vi "Main.vi"() -> ()   [LabVIEW 2018] (continued)
                n2991 = call "S7_Read.vi"("TCP"=w2079, "DB #"=u16 20, "读取长度"=u16 13, "寄存器类型"=w2083, "起始地址"=u32 82, "数据类型"=w2081, "error in"=w2078) -> ("TCP"=w2077:refnum<k5>, "数据"=w2086:u32[], "error out"=w2088:errorcluster)  [unwired: 5 in, 1 out]
                n2992 = To Unsigned Word Integer(number=w2086) -> (unsigned 16bit integer=w2087:u16[])
                n2993 = call "还原为字符串.vi"("error in (no error)"=w2088, "输入数组"=w2087) -> ("error out"=w2076:errorcluster, "字符串"=w2080:string)  [unwired: 8 in]
                n2994 = call "S7_Read.vi"("TCP"=w2077, "DB #"=u16 20, "读取长度"=u16 2, "寄存器类型"=w2105, "起始地址"=u32 212, "数据类型"=w2107, "error in"=w2076) -> ("TCP"=w2101:refnum<k5>, "数据"=w2100:u32[], "error out"=w2102:errorcluster)  [unwired: 5 in, 1 out]
                n2995 = Index Array(array=w2100) -> (element #1=w2099:u32, element #2=w2095:u32)  [unwired: 2 in]
                n2996 = Equal?(x=w2095, y=u32 1) -> (x = y?=w2096:bool)
                n2997 = Equal?(x=w2099, y=u32 1) -> (x = y?=w2094:bool)
                n2998 = call "S7_Read.vi"("TCP"=w2101, "DB #"=u16 20, "读取长度"=u16 1, "寄存器类型"=w2111, "起始地址"=u32 136, "数据类型"=w2109, "error in"=w2102) -> ("TCP"=w2125:refnum<k5>, "数据"=w2127:u32[], "error out"=w2126:errorcluster)  [unwired: 5 in, 1 out]
                n2999 = case shown="真" w2096 {
                  tunnel: ["NG" "OK"] -> w2092
                  frame False {
                  }
                  frame True {
                  }
                }
                n3000 = case shown="真" w2094 {
                  tunnel: ["NG" "OK"] -> w2093
                  frame False {
                  }
                  frame True {
                  }
                }
                n3001 = local write "503二维码"(w2080) -> ()
                n3002 = call "S7_Read.vi"("TCP"=w2125, "DB #"=u16 20, "读取长度"=u16 1, "寄存器类型"=w2116, "起始地址"=u32 128, "数据类型"=w2114, "error in"=w2126) -> ("TCP"=w2108:refnum<k5>, "数据"=w2129:u32[], "error out"=w2091:errorcluster)  [unwired: 5 in, 1 out]
                n3003 = Index Array(array=w2127) -> (element=w2128:u32)  [unwired: 1 in]
                n3004 = Number To Decimal String(number=w2128) -> (decimal integer string=w2135:string)  [unwired: 1 in]
                n3005 = Index Array(array=w2129) -> (element=w2131:u32)  [unwired: 1 in]
                n3006 = Equal?(x=w2131, y=u32 1) -> (x = y?=w2130:bool)
                n3007 = case shown="真" w2130 {
                  tunnel: ["NG" "OK"] -> w2134
                  frame False {
                  }
                  frame True {
                  }
                }
                n3008 = Format Date/Time String(time format string (%c)="%Y-%m-%d" ("时间格式字符串(%c)")) -> (date/time string=w2132:string)  [unwired: 2 in]
                n3009 = Get Date/Time String(want seconds? (F)=TRUE ("需要秒？(F)")) -> (time string=w2133:string)  [unwired: 2 in, 1 out]
                n3010 = Insert Into Array(array=string[] [] ("数组"), index=0 ("索引"), new element #1="503" ("新元素/子数组"), new element #2=w2134, new element #3=w2132, new element #4=w2133, new element #5=w2134, new element #6=w2135, new element #7=w2093, new element #8=w2092) -> (w2089:string[])
                n3011 = stacked-sequence {
                  tunnel: w2091 -> [_ w2139]
                  tunnel: [_ w2138] -> w2090
                  tunnel: w2089 -> [w2136 _]
                  frame #0 {
                    "503data" <- w2136
                  }
                  frame #1 {
                    n3012 = property on="ST503数据读取（事件）" class="Bool (严格)"(error in=w2139, "Val(Sgnl)"=TRUE ("值(信号)")) -> (error out=w2138:errorcluster)  [unwired: 1 in, 1 out]
                  }
                }
              }
            }
            n3013 = call <vilib>:"Boolean Crossing PtByPt.vi"("direction"=enum16{"either", "false-true", "true-false"}."false-true", "input"=w1819) -> ("crossing"=w1830:bool)  [unwired: 1 in]
            n3014 = case shown="真" w1830 {
              tunnel: w1829 -> [w2052 w2058]
              tunnel: w1828 -> [w2051 w2057]
              tunnel: [w2051 w2054] -> w1827
              tunnel: [w2052 w2056] -> w1826
              frame False {
              }
              frame True {
                w2059 = u16 0 items=["byte", "word", "Dword"] ("数据类型")
                w2061 = u8 132 items=["I/O (P)"=128, "Input (I)"=129, "Output (Q)"=130, "Bit Memory (M)"=131, "Data (DB)"=132, "Instance Data (DI)"=133, "Local Data (L)"=134, "Predecessor Local Data (VL)"=135] ("寄存器类型")
                # "原82"
                n3015 = call "S7_Read.vi"("TCP"=w2058, "DB #"=u16 20, "读取长度"=u16 13, "寄存器类型"=w2061, "起始地址"=u32 104, "数据类型"=w2059, "error in"=w2057) -> ("TCP"=w2056:refnum<k5>, "数据"=w2064:u32[], "error out"=w2066:errorcluster)  [unwired: 5 in, 1 out]
                n3016 = To Unsigned Word Integer(number=w2064) -> (unsigned 16bit integer=w2065:u16[])
                n3017 = call "还原为字符串.vi"("error in (no error)"=w2066, "输入数组"=w2065) -> ("error out"=w2055:errorcluster, "字符串"=w2053:string)  [unwired: 8 in]
                n3018 = stacked-sequence {
                  tunnel: w2055 -> [_ w2070]
                  tunnel: [_ w2069] -> w2054
                  tunnel: w2053 -> [w2067 _]
                  frame #0 {
                    "504二维码" <- w2067
                  }
                  frame #1 {
                    n3019 = property on="ST504扫码请求（事件）" class="Bool (严格)"(error in=w2070, "Val(Sgnl)"=TRUE ("值(信号)")) -> (error out=w2069:errorcluster)  [unwired: 1 in, 1 out]
                  }
                }
              }
            }
            n3020 = call <vilib>:"Boolean Crossing PtByPt.vi"("direction"=enum16{"either", "false-true", "true-false"}."false-true", "input"=w1818) -> ("crossing"=w1824:bool)  [unwired: 1 in]
            n3021 = case shown="真" w1824 {
              tunnel: w1826 -> [w1919 w1923]
              tunnel: w1827 -> [w1918 w1922]
              tunnel: [w1919 w2009] -> w1823
              tunnel: [w1918 w1934] -> w1822
              frame False {
              }
              frame True {
                w1925 = u16 0 items=["byte", "word", "Dword"] ("数据类型")
                w1927 = u8 132 items=["I/O (P)"=128, "Input (I)"=129, "Output (Q)"=130, "Bit Memory (M)"=131, "Data (DB)"=132, "Instance Data (DI)"=133, "Local Data (L)"=134, "Predecessor Local Data (VL)"=135] ("寄存器类型")
                w1970 = 15 ("长度")
                w1980 = u16 0 items=["byte", "word", "Dword"] ("数据类型")
                w1982 = u8 132 items=["I/O (P)"=128, "Input (I)"=129, "Output (Q)"=130, "Bit Memory (M)"=131, "Data (DB)"=132, "Instance Data (DI)"=133, "Local Data (L)"=134, "Predecessor Local Data (VL)"=135] ("寄存器类型")
                w2008 = u16 1 items=["byte", "word", "Dword"] ("数据类型")
                w2006 = u8 132 items=["I/O (P)"=128, "Input (I)"=129, "Output (Q)"=130, "Bit Memory (M)"=131, "Data (DB)"=132, "Instance Data (DI)"=133, "Local Data (L)"=134, "Predecessor Local Data (VL)"=135] ("寄存器类型")
                w2015 = u16 1 items=["byte", "word", "Dword"] ("数据类型")
                w2017 = u8 132 items=["I/O (P)"=128, "Input (I)"=129, "Output (Q)"=130, "Bit Memory (M)"=131, "Data (DB)"=132, "Instance Data (DI)"=133, "Local Data (L)"=134, "Predecessor Local Data (VL)"=135] ("寄存器类型")
                w2010 = u16 1 items=["byte", "word", "Dword"] ("数据类型")
                w2012 = u8 132 items=["I/O (P)"=128, "Input (I)"=129, "Output (Q)"=130, "Bit Memory (M)"=131, "Data (DB)"=132, "Instance Data (DI)"=133, "Local Data (L)"=134, "Predecessor Local Data (VL)"=135] ("寄存器类型")
                n3022 = call "S7_Read.vi"("TCP"=w1923, "DB #"=u16 20, "读取长度"=u16 13, "寄存器类型"=w1927, "起始地址"=u32 104, "数据类型"=w1925, "error in"=w1922) -> ("TCP"=w1921:refnum<k5>, "数据"=w1930:u32[], "error out"=w1932:errorcluster)  [unwired: 5 in, 1 out]
                n3023 = To Unsigned Word Integer(number=w1930) -> (unsigned 16bit integer=w1931:u16[])
                n3024 = call "还原为字符串.vi"("error in (no error)"=w1932, "输入数组"=w1931) -> ("error out"=w1920:errorcluster, "字符串"=w1924:string)  [unwired: 8 in]
                n3025 = call "S7_Read.vi"("TCP"=w1921, "DB #"=u16 20, "读取长度"=u16 105, "寄存器类型"=w1982, "起始地址"=u32 224, "数据类型"=w1980, "error in"=w1920) -> ("TCP"=w1979:refnum<k5>, "数据"=w1972:u32[], "error out"=w1978:errorcluster)  [unwired: 5 in, 1 out]
                n3026 = Delete From Array(array=w1972, length=w1970, index=2 ("索引")) -> (deleted portion=w1971:u32[])  [unwired: 1 out]
                n3027 = Delete From Array(array=w1972, length=w1970, index=22 ("索引")) -> (deleted portion=w1943:u32[])  [unwired: 1 out]
                n3028 = Delete From Array(array=w1972, length=w1970, index=42 ("索引")) -> (deleted portion=w1942:u32[])  [unwired: 1 out]
                n3029 = Delete From Array(array=w1972, length=w1970, index=62 ("索引")) -> (deleted portion=w1941:u32[])  [unwired: 1 out]
                n3030 = Delete From Array(array=w1972, length=w1970, index=82 ("索引")) -> (deleted portion=w1940:u32[])  [unwired: 1 out]
                n3031 = local write "504二维码"(w1924) -> ()
                n3032 = To Unsigned Word Integer(number=w1943) -> (unsigned 16bit integer=w1959:u16[])
                n3033 = To Unsigned Word Integer(number=w1941) -> (unsigned 16bit integer=w1958:u16[])
                n3034 = To Unsigned Word Integer(number=w1971) -> (unsigned 16bit integer=w1977:u16[])
                n3035 = To Unsigned Word Integer(number=w1940) -> (unsigned 16bit integer=w1944:u16[])
                n3036 = call "S7_Read.vi"("TCP"=w1979, "DB #"=u16 20, "读取长度"=u16 4, "寄存器类型"=w2006, "起始地址"=u32 216, "数据类型"=w2008, "error in"=w1978) -> ("TCP"=w2002:refnum<k5>, "数据"=w2001:u32[], "error out"=w2003:errorcluster)  [unwired: 5 in, 1 out]
                n3037 = To Unsigned Word Integer(number=w1942) -> (unsigned 16bit integer=w1949:u16[])
                n3038 = call "还原为字符串.vi"("输入数组"=w1977) -> ("字符串"=w1975:string)  [unwired: 9 in, 1 out]
                n3039 = call "还原为字符串.vi"("输入数组"=w1959) -> ("字符串"=w1961:string)  [unwired: 9 in, 1 out]
                n3040 = call "还原为字符串.vi"("输入数组"=w1949) -> ("字符串"=w1951:string)  [unwired: 9 in, 1 out]
                n3041 = call "还原为字符串.vi"("输入数组"=w1958) -> ("字符串"=w1956:string)  [unwired: 9 in, 1 out]
                n3042 = call "还原为字符串.vi"("输入数组"=w1944) -> ("字符串"=w1946:string)  [unwired: 9 in, 1 out]
                n3043 = Index Array(array=w2001) -> (element #1=w2000:u32, element #2=w1996:u32, element #3=w1988:u32, element #4=w1987:u32)  [unwired: 4 in]
                n3044 = Match Pattern(string=w1975, regular expression="\r" ("正则表达式")) -> (before substring=w1976:string)  [unwired: 1 in, 3 out]
                n3045 = Match Pattern(string=w1961, regular expression="\r" ("正则表达式")) -> (before substring=w1960:string)  [unwired: 1 in, 3 out]
                n3046 = Match Pattern(string=w1951, regular expression="\r" ("正则表达式")) -> (before substring=w1950:string)  [unwired: 1 in, 3 out]
                n3047 = Match Pattern(string=w1956, regular expression="\r" ("正则表达式")) -> (before substring=w1957:string)  [unwired: 1 in, 3 out]
                n3048 = Match Pattern(string=w1946, regular expression="\r" ("正则表达式")) -> (before substring=w1945:string)  [unwired: 1 in, 3 out]
                n3049 = Equal?(x=w1987, y=u32 1) -> (x = y?=w1991:bool)
                n3050 = Equal?(x=w1996, y=u32 1) -> (x = y?=w1997:bool)
                n3051 = Equal?(x=w1988, y=u32 1) -> (x = y?=w1992:bool)
                n3052 = Equal?(x=w2000, y=u32 1) -> (x = y?=w1995:bool)
                n3053 = call "S7_Read.vi"("TCP"=w2002, "DB #"=u16 20, "读取长度"=u16 1, "寄存器类型"=w2012, "起始地址"=u32 138, "数据类型"=w2010, "error in"=w2003) -> ("TCP"=w2026:refnum<k5>, "数据"=w2028:u32[], "error out"=w2027:errorcluster)  [unwired: 5 in, 1 out]
                n3054 = case shown="真" w1991 {
                  tunnel: ["NG" "OK"] -> w1985
                  frame False {
                  }
                  frame True {
                  }
                }
                n3055 = case shown="真" w1997 {
                  tunnel: ["NG" "OK"] -> w1993
                  frame False {
                  }
                  frame True {
                  }
                }
                n3056 = case shown="真" w1992 {
                  tunnel: ["NG" "OK"] -> w1986
                  frame False {
                  }
                  frame True {
                  }
                }
                n3057 = case shown="真" w1995 {
                  tunnel: ["NG" "OK"] -> w1994
                  frame False {
                  }
                  frame True {
                  }
                }
                n3058 = Match Pattern(string=w1976, regular expression="\u0000" ("正则表达式")) -> (before substring=w1964:string)  [unwired: 1 in, 3 out]
                n3059 = Match Pattern(string=w1960, regular expression="\u0000" ("正则表达式")) -> (before substring=w1939:string)  [unwired: 1 in, 3 out]
                n3060 = Match Pattern(string=w1950, regular expression="\u0000" ("正则表达式")) -> (before substring=w1938:string)  [unwired: 1 in, 3 out]
                n3061 = Match Pattern(string=w1957, regular expression="\u0000" ("正则表达式")) -> (before substring=w1937:string)  [unwired: 1 in, 3 out]
                n3062 = Match Pattern(string=w1945, regular expression="\u0000" ("正则表达式")) -> (before substring=w1936:string)  [unwired: 1 in, 3 out]
                n3063 = Index Array(array=w2028) -> (element=w2029:u32)  [unwired: 1 in]
                n3064 = call "S7_Read.vi"("TCP"=w2026, "DB #"=u16 20, "读取长度"=u16 1, "寄存器类型"=w2017, "起始地址"=u32 130, "数据类型"=w2015, "error in"=w2027) -> ("TCP"=w2009:refnum<k5>, "数据"=w2030:u32[], "error out"=w1935:errorcluster)  [unwired: 5 in, 1 out]
                n3065 = Number To Decimal String(number=w2029) -> (decimal integer string=w2036:string)  [unwired: 1 in]
                n3066 = Index Array(array=w2030) -> (element=w2032:u32)  [unwired: 1 in]
                n3067 = Equal?(x=w2032, y=u32 1) -> (x = y?=w2031:bool)
                n3068 = case shown="真" w2031 {
                  tunnel: ["NG" "OK"] -> w2035
                  frame False {
                  }
                  frame True {
                  }
                }
                n3069 = Format Date/Time String(time format string (%c)="%Y-%m-%d" ("时间格式字符串(%c)")) -> (date/time string=w2033:string)  [unwired: 2 in]
                n3070 = Get Date/Time String(want seconds? (F)=TRUE ("需要秒？(F)")) -> (time string=w2034:string)  [unwired: 2 in, 1 out]
                n3071 = Insert Into Array(array=string[] [] ("数组"), index=0 ("索引"), new element #1="504" ("新元素/子数组"), new element #2=w2035, new element #3=w2033, new element #4=w2034, new element #5=w2035, new element #6=w2036, new element #7=w1994, new element #8=w1993, new element #9=w1986, new element #10=w1985, new element #11=w1964, new element #12=w1939, new element #13=w1938, new element #14=w1937, new element #15=w1936) -> (w1933:string[])
                n3072 = stacked-sequence {
                  tunnel: w1935 -> [_ w2040]
                  tunnel: [_ w2039] -> w1934
                  tunnel: w1933 -> [w2037 _]
                  frame #0 {
                    "504data" <- w2037
                  }
                  frame #1 {
                    n3073 = property on="ST504数据读取（事件）" class="Bool (严格)"(error in=w2040, "Val(Sgnl)"=TRUE ("值(信号)")) -> (error out=w2039:errorcluster)  [unwired: 1 in, 1 out]
                  }
                }
              }
            }
          }
          frame "写" {
            w2399 = u8 132 items=["I/O (P)"=128, "Input (I)"=129, "Output (Q)"=130, "Bit Memory (M)"=131, "Data (DB)"=132, "Instance Data (DI)"=133, "Local Data (L)"=134, "Predecessor Local Data (VL)"=135] ("寄存器类型")
            w2400 = u16 1 items=["byte", "word", "Dword"] ("数据类型")
            w2406 = u8 132 items=["I/O (P)"=128, "Input (I)"=129, "Output (Q)"=130, "Bit Memory (M)"=131, "Data (DB)"=132, "Instance Data (DI)"=133, "Local Data (L)"=134, "Predecessor Local Data (VL)"=135] ("寄存器类型")
            w2407 = u16 1 items=["byte", "word", "Dword"] ("数据类型")
            w2420 = u8 132 items=["I/O (P)"=128, "Input (I)"=129, "Output (Q)"=130, "Bit Memory (M)"=131, "Data (DB)"=132, "Instance Data (DI)"=133, "Local Data (L)"=134, "Predecessor Local Data (VL)"=135] ("寄存器类型")
            w2419 = u16 1 items=["byte", "word", "Dword"] ("数据类型")
            w2413 = u8 132 items=["I/O (P)"=128, "Input (I)"=129, "Output (Q)"=130, "Bit Memory (M)"=131, "Data (DB)"=132, "Instance Data (DI)"=133, "Local Data (L)"=134, "Predecessor Local Data (VL)"=135] ("寄存器类型")
            w2412 = u16 1 items=["byte", "word", "Dword"] ("数据类型")
            w2438 = u8 132 items=["I/O (P)"=128, "Input (I)"=129, "Output (Q)"=130, "Bit Memory (M)"=131, "Data (DB)"=132, "Instance Data (DI)"=133, "Local Data (L)"=134, "Predecessor Local Data (VL)"=135] ("寄存器类型")
            w2437 = u16 1 items=["byte", "word", "Dword"] ("数据类型")
            w2451 = u8 132 items=["I/O (P)"=128, "Input (I)"=129, "Output (Q)"=130, "Bit Memory (M)"=131, "Data (DB)"=132, "Instance Data (DI)"=133, "Local Data (L)"=134, "Predecessor Local Data (VL)"=135] ("寄存器类型")
            w2452 = u16 1 items=["byte", "word", "Dword"] ("数据类型")
            w2458 = u8 132 items=["I/O (P)"=128, "Input (I)"=129, "Output (Q)"=130, "Bit Memory (M)"=131, "Data (DB)"=132, "Instance Data (DI)"=133, "Local Data (L)"=134, "Predecessor Local Data (VL)"=135] ("寄存器类型")
            w2459 = u16 1 items=["byte", "word", "Dword"] ("数据类型")
            w2461 = u8 132 items=["I/O (P)"=128, "Input (I)"=129, "Output (Q)"=130, "Bit Memory (M)"=131, "Data (DB)"=132, "Instance Data (DI)"=133, "Local Data (L)"=134, "Predecessor Local Data (VL)"=135] ("寄存器类型")
            w2460 = u16 1 items=["byte", "word", "Dword"] ("数据类型")
            w2468 = u8 132 items=["I/O (P)"=128, "Input (I)"=129, "Output (Q)"=130, "Bit Memory (M)"=131, "Data (DB)"=132, "Instance Data (DI)"=133, "Local Data (L)"=134, "Predecessor Local Data (VL)"=135] ("寄存器类型")
            w2465 = u16 1 items=["byte", "word", "Dword"] ("数据类型")
            n3074 = local read "50看门狗"() -> (w2431:i32)
            n3075 = case shown="0" w2431 {
              tunnel: [0 ("y") 1 ("y")] -> w2430
              frame 1, Default {
              }
              frame 0 {
              }
            }
            "50看门狗" <- w2430
            n3076 = call "S7_Write.vi"("TCP"=w2464, "寄存器类型"=w2468, "DB #"=u16 20, "写入地址"=u32 2, "数据类型"=w2465, "写入数据"=w2430) -> ("TCP"=w2445:refnum<k5>, "error out"=w2444:errorcluster)  [unwired: 7 in, 1 out]
            n3077 = case shown="假" "501扫码回复输入" {
              tunnel: w2445 -> [w2547 w2555]
              tunnel: w2444 -> [w2546 w2554]
              tunnel: [w2547 w2553] -> w2443
              tunnel: [w2546 w2552] -> w2442
              tunnel: [999 w2551] -> w2441
              frame False {
              }
              frame True {
                w2563 = u8 132 items=["I/O (P)"=128, "Input (I)"=129, "Output (Q)"=130, "Bit Memory (M)"=131, "Data (DB)"=132, "Instance Data (DI)"=133, "Local Data (L)"=134, "Predecessor Local Data (VL)"=135] ("寄存器类型")
                w2562 = u16 1 items=["byte", "word", "Dword"] ("数据类型")
                w2557 = u8 132 items=["I/O (P)"=128, "Input (I)"=129, "Output (Q)"=130, "Bit Memory (M)"=131, "Data (DB)"=132, "Instance Data (DI)"=133, "Local Data (L)"=134, "Predecessor Local Data (VL)"=135] ("寄存器类型")
                w2558 = u16 1 items=["byte", "word", "Dword"] ("数据类型")
                n3078 = local read "上一站号 (501)"() -> (w2550:string)
                n3079 = local read "上一站结果 (501)"() -> (w2549:string)
                n3080 = Decimal String To Number(string=w2550, default (0L)=u32 0 ("默认(0 I32)")) -> (number=w2567:u32)  [unwired: 1 in, 1 out]
                n3081 = call "S7_Write.vi"("TCP"=w2555, "寄存器类型"=w2557, "DB #"=u16 20, "写入地址"=u32 20, "数据类型"=w2558, "写入数据"=w2567, "error in"=w2554) -> ("TCP"=w2566:refnum<k5>, "error out"=w2565:errorcluster)  [unwired: 6 in, 1 out]
                n3082 = Equal?(x=w2549, y="OK") -> (x = y?=w2569:bool)
                n3083 = case shown="真" w2569 {
                  tunnel: [u32 2 ("写入数据") u32 1 ("写入数据")] -> w2570
                  frame False {
                  }
                  frame True {
                  }
                }
                n3084 = local read "扫码请求回复501"() -> (w2548:string)
                n3085 = call "S7_Write.vi"("TCP"=w2566, "寄存器类型"=w2563, "DB #"=u16 20, "写入地址"=u32 22, "数据类型"=w2562, "写入数据"=w2570, "error in"=w2565) -> ("TCP"=w2553:refnum<k5>, "error out"=w2552:errorcluster)  [unwired: 6 in, 1 out]
                n3086 = Decimal String To Number(string=w2548) -> (number=w2551:i32)  [unwired: 2 in, 1 out]
              }
            }
            n3087 = call "S7_Write.vi"("TCP"=w2443, "寄存器类型"=w2461, "DB #"=u16 20, "写入地址"=u32 4, "数据类型"=w2460, "写入数据"=w2441, "error in"=w2442) -> ("TCP"=w2436:refnum<k5>, "error out"=w2435:errorcluster)  [unwired: 6 in, 1 out]
            n3088 = case shown="真" "501数据回复输入" {
              tunnel: [999 w2544] -> w2434
              frame False {
              }
              frame True {
                n3089 = local read "数据保存请求回复501"() -> (w2543:string)
                n3090 = Decimal String To Number(string=w2543) -> (number=w2544:i32)  [unwired: 2 in, 1 out]
              }
            }
            n3091 = call "S7_Write.vi"("TCP"=w2436, "寄存器类型"=w2438, "DB #"=u16 20, "写入地址"=u32 6, "数据类型"=w2437, "写入数据"=w2434, "error in"=w2435) -> ("TCP"=w2433:refnum<k5>, "error out"=w2432:errorcluster)  [unwired: 6 in, 1 out]
            n3092 = case shown="假" "502扫码回复输入" {
              tunnel: [999 w2582] -> w2455
              tunnel: w2433 -> [w2577 w2596]
              tunnel: w2432 -> [w2576 w2595]
              tunnel: [w2577 w2584] -> w2454
              tunnel: [w2576 w2583] -> w2453
              frame False {
              }
              frame True {
                w2590 = u8 132 items=["I/O (P)"=128, "Input (I)"=129, "Output (Q)"=130, "Bit Memory (M)"=131, "Data (DB)"=132, "Instance Data (DI)"=133, "Local Data (L)"=134, "Predecessor Local Data (VL)"=135] ("寄存器类型")
                w2591 = u16 1 items=["byte", "word", "Dword"] ("数据类型")
                w2598 = u8 132 items=["I/O (P)"=128, "Input (I)"=129, "Output (Q)"=130, "Bit Memory (M)"=131, "Data (DB)"=132, "Instance Data (DI)"=133, "Local Data (L)"=134, "Predecessor Local Data (VL)"=135] ("寄存器类型")
                w2597 = u16 1 items=["byte", "word", "Dword"] ("数据类型")
                n3093 = local read "上一站号 (502)"() -> (w2581:string)
                n3094 = Decimal String To Number(string=w2581) -> (number=w2594:i32)  [unwired: 2 in, 1 out]
                n3095 = call "S7_Write.vi"("TCP"=w2596, "寄存器类型"=w2598, "DB #"=u16 20, "写入地址"=u32 24, "数据类型"=w2597, "写入数据"=w2594, "error in"=w2595) -> ("TCP"=w2586:refnum<k5>, "error out"=w2587:errorcluster)  [unwired: 6 in, 1 out]
                n3096 = local read "上一站结果 (502)"() -> (w2580:string)
                n3097 = local read "扫码请求回复502"() -> (w2579:string)
                n3098 = Equal?(x=w2580, y="OK") -> (x = y?=w2593:bool)
                n3099 = case shown="假" w2593 {
                  tunnel: [u32 2 ("写入数据") u32 1 ("写入数据")] -> w2585
                  frame False {
                  }
                  frame True {
                  }
                }
                n3100 = call "S7_Write.vi"("TCP"=w2586, "寄存器类型"=w2590, "DB #"=u16 20, "写入地址"=u32 26, "数据类型"=w2591, "写入数据"=w2585, "error in"=w2587) -> ("TCP"=w2584:refnum<k5>, "error out"=w2583:errorcluster)  [unwired: 6 in, 1 out]
                n3101 = Decimal String To Number(string=w2579) -> (number=w2582:i32)  [unwired: 2 in, 1 out]
              }
            }
            n3102 = call "S7_Write.vi"("TCP"=w2454, "寄存器类型"=w2458, "DB #"=u16 20, "写入地址"=u32 8, "数据类型"=w2459, "写入数据"=w2455, "error in"=w2453) -> ("TCP"=w2447:refnum<k5>, "error out"=w2448:errorcluster)  [unwired: 6 in, 1 out]
            n3103 = case shown="真" "502数据回复输入" {
              tunnel: [999 w2575] -> w2446
              frame False {
              }
              frame True {
                n3104 = local read "数据保存请求回复502"() -> (w2574:string)
                n3105 = Decimal String To Number(string=w2574) -> (number=w2575:i32)  [unwired: 2 in, 1 out]
              }
            }
            n3106 = call "S7_Write.vi"("TCP"=w2447, "寄存器类型"=w2451, "DB #"=u16 20, "写入地址"=u32 10, "数据类型"=w2452, "写入数据"=w2446, "error in"=w2448) -> ("TCP"=w2411:refnum<k5>, "error out"=w2410:errorcluster)  [unwired: 6 in, 1 out]
            n3107 = case shown="假" "503扫码回复输入" {
              tunnel: [999 w2521] -> w2416
              tunnel: w2411 -> [w2516 w2535]
              tunnel: w2410 -> [w2515 w2534]
              tunnel: [w2516 w2523] -> w2417
              tunnel: [w2515 w2522] -> w2418
              frame False {
              }
              frame True {
                w2529 = u8 132 items=["I/O (P)"=128, "Input (I)"=129, "Output (Q)"=130, "Bit Memory (M)"=131, "Data (DB)"=132, "Instance Data (DI)"=133, "Local Data (L)"=134, "Predecessor Local Data (VL)"=135] ("寄存器类型")
                w2530 = u16 1 items=["byte", "word", "Dword"] ("数据类型")
                w2537 = u8 132 items=["I/O (P)"=128, "Input (I)"=129, "Output (Q)"=130, "Bit Memory (M)"=131, "Data (DB)"=132, "Instance Data (DI)"=133, "Local Data (L)"=134, "Predecessor Local Data (VL)"=135] ("寄存器类型")
                w2536 = u16 1 items=["byte", "word", "Dword"] ("数据类型")
                n3108 = local read "上一站号 (503)"() -> (w2520:string)
                n3109 = Decimal String To Number(string=w2520) -> (number=w2533:i32)  [unwired: 2 in, 1 out]
                n3110 = call "S7_Write.vi"("TCP"=w2535, "寄存器类型"=w2537, "DB #"=u16 20, "写入地址"=u32 28, "数据类型"=w2536, "写入数据"=w2533, "error in"=w2534) -> ("TCP"=w2525:refnum<k5>, "error out"=w2526:errorcluster)  [unwired: 6 in, 1 out]
                n3111 = local read "上一站结果 (503)"() -> (w2519:string)
                n3112 = local read "扫码请求回复503"() -> (w2518:string)
                n3113 = Equal?(x=w2519, y="OK") -> (x = y?=w2532:bool)
                n3114 = case shown="假" w2532 {
                  tunnel: [u32 2 ("写入数据") u32 1 ("写入数据")] -> w2524
                  frame False {
                  }
                  frame True {
                  }
                }
                n3115 = call "S7_Write.vi"("TCP"=w2525, "寄存器类型"=w2529, "DB #"=u16 20, "写入地址"=u32 30, "数据类型"=w2530, "写入数据"=w2524, "error in"=w2526) -> ("TCP"=w2523:refnum<k5>, "error out"=w2522:errorcluster)  [unwired: 6 in, 1 out]
                n3116 = Decimal String To Number(string=w2518) -> (number=w2521:i32)  [unwired: 2 in, 1 out]
              }
            }
            n3117 = call "S7_Write.vi"("TCP"=w2417, "寄存器类型"=w2413, "DB #"=u16 20, "写入地址"=u32 12, "数据类型"=w2412, "写入数据"=w2416, "error in"=w2418) -> ("TCP"=w2424:refnum<k5>, "error out"=w2423:errorcluster)  [unwired: 6 in, 1 out]
            n3118 = case shown="真" "503数据回复输入" {
              tunnel: [999 w2514] -> w2425
              frame False {
              }
              frame True {
                n3119 = local read "数据保存请求回复503"() -> (w2513:string)
                n3120 = Decimal String To Number(string=w2513) -> (number=w2514:i32)  [unwired: 2 in, 1 out]
              }
            }
            n3121 = call "S7_Write.vi"("TCP"=w2424, "寄存器类型"=w2420, "DB #"=u16 20, "写入地址"=u32 14, "数据类型"=w2419, "写入数据"=w2425, "error in"=w2423) -> ("TCP"=w2393:refnum<k5>, "error out"=w2392:errorcluster)  [unwired: 6 in, 1 out]
            n3122 = case shown="假" "504扫码回复输入" {
              tunnel: [999 w2491] -> w2403
              tunnel: w2393 -> [w2486 w2505]
              tunnel: w2392 -> [w2485 w2504]
              tunnel: [w2486 w2493] -> w2402
              tunnel: [w2485 w2492] -> w2401
              frame False {
              }
              frame True {
                w2499 = u8 132 items=["I/O (P)"=128, "Input (I)"=129, "Output (Q)"=130, "Bit Memory (M)"=131, "Data (DB)"=132, "Instance Data (DI)"=133, "Local Data (L)"=134, "Predecessor Local Data (VL)"=135] ("寄存器类型")
                w2500 = u16 1 items=["byte", "word", "Dword"] ("数据类型")
                w2507 = u8 132 items=["I/O (P)"=128, "Input (I)"=129, "Output (Q)"=130, "Bit Memory (M)"=131, "Data (DB)"=132, "Instance Data (DI)"=133, "Local Data (L)"=134, "Predecessor Local Data (VL)"=135] ("寄存器类型")
                w2506 = u16 1 items=["byte", "word", "Dword"] ("数据类型")
                n3123 = local read "上一站号 (504)"() -> (w2490:string)
                n3124 = Decimal String To Number(string=w2490) -> (number=w2503:i32)  [unwired: 2 in, 1 out]
                n3125 = call "S7_Write.vi"("TCP"=w2505, "寄存器类型"=w2507, "DB #"=u16 20, "写入地址"=u32 32, "数据类型"=w2506, "写入数据"=w2503, "error in"=w2504) -> ("TCP"=w2495:refnum<k5>, "error out"=w2496:errorcluster)  [unwired: 6 in, 1 out]
                n3126 = local read "上一站结果 (504)"() -> (w2489:string)
                n3127 = local read "扫码请求回复504"() -> (w2488:string)
                n3128 = Equal?(x=w2489, y="OK") -> (x = y?=w2502:bool)
                n3129 = case shown="假" w2502 {
                  tunnel: [u32 2 ("写入数据") u32 1 ("写入数据")] -> w2494
                  frame False {
                  }
                  frame True {
                  }
                }
                n3130 = call "S7_Write.vi"("TCP"=w2495, "寄存器类型"=w2499, "DB #"=u16 20, "写入地址"=u32 34, "数据类型"=w2500, "写入数据"=w2494, "error in"=w2496) -> ("TCP"=w2493:refnum<k5>, "error out"=w2492:errorcluster)  [unwired: 6 in, 1 out]
                n3131 = Decimal String To Number(string=w2488) -> (number=w2491:i32)  [unwired: 2 in, 1 out]
              }
            }
            n3132 = call "S7_Write.vi"("TCP"=w2402, "寄存器类型"=w2406, "DB #"=u16 20, "写入地址"=u32 16, "数据类型"=w2407, "写入数据"=w2403, "error in"=w2401) -> ("TCP"=w2395:refnum<k5>, "error out"=w2396:errorcluster)  [unwired: 6 in, 1 out]
            n3133 = case shown="真" "504数据回复输入" {
              tunnel: [999 w2484] -> w2394
              frame False {
              }
              frame True {
                n3134 = local read "数据保存请求回复504"() -> (w2483:string)
                n3135 = Decimal String To Number(string=w2483) -> (number=w2484:i32)  [unwired: 2 in, 1 out]
              }
            }
            n3136 = call "S7_Write.vi"("TCP"=w2395, "寄存器类型"=w2399, "DB #"=u16 20, "写入地址"=u32 18, "数据类型"=w2400, "写入数据"=w2394, "error in"=w2396) -> ("TCP"=w2389:refnum<k5>, "error out"=w2387:errorcluster)  [unwired: 6 in, 1 out]
            n3137 = disable-structure shown="启用" {
              disable-tunnel: w2389 -> [w2471 w2475]
              disable-tunnel: [w2471 w2478] -> w2388
              disable-tunnel: w2387 -> [w2472 w2476]
              disable-tunnel: [w2472 w2477] -> w2386
              frame Disabled {
              }
              frame Enabled {
                w2480 = u8 132 items=["I/O (P)"=128, "Input (I)"=129, "Output (Q)"=130, "Bit Memory (M)"=131, "Data (DB)"=132, "Instance Data (DI)"=133, "Local Data (L)"=134, "Predecessor Local Data (VL)"=135] ("寄存器类型")
                w2474 = u16 1 items=["byte", "word", "Dword"] ("数据类型")
                n3138 = local read "产品型号"() -> (w2473:u32)
                n3139 = call "S7_Write.vi"("TCP"=w2475, "寄存器类型"=w2480, "DB #"=u16 20, "写入地址"=u32 324, "数据类型"=w2474, "写入数据"=w2473, "error in"=w2476) -> ("TCP"=w2478:refnum<k5>, "error out"=w2477:errorcluster)  [unwired: 6 in, 1 out]
              }
            }
          }
          frame "错误" {
            n3140 = call "S7_Close.vi"("TCP Connection Ref"=w2607) -> ("error out"=w2608:errorcluster)  [unwired: 10 in]
            n3141 = call <vilib>:"Clear Errors.vi"("error in (no error)"=w2608) -> ()  [unwired: 5 in, 2 out]
          }
          frame "退出" {
            n3142 = call "S7_Close.vi"("TCP Connection Ref"=w2614) -> ("error out"=w2615:errorcluster)  [unwired: 10 in]
            n3143 = call <vilib>:"Clear Errors.vi"("error in (no error)"=w2615) -> ()  [unwired: 5 in, 2 out]
          }
        }
      }
    }
  }
